vi "BallShear_BallShear.vi"(8 "Check":bool, 10 "Speed":dbl, 11 "Selected Balls":dbl[][](array[numeric])) -> (0 "Ready":bool, 3 "Status":string)   [LabVIEW 2013]
panel:
  in  "Y Val":dbl
  in  "X Val":dbl
  out "Selected Balls 2":dbl[][](array[numeric])
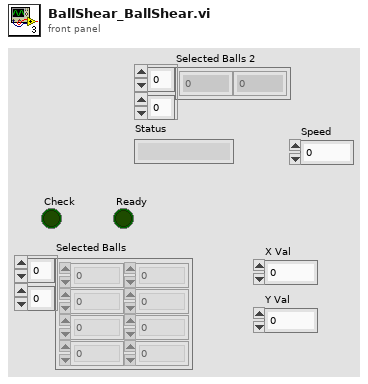
[diagram p1: front panel]
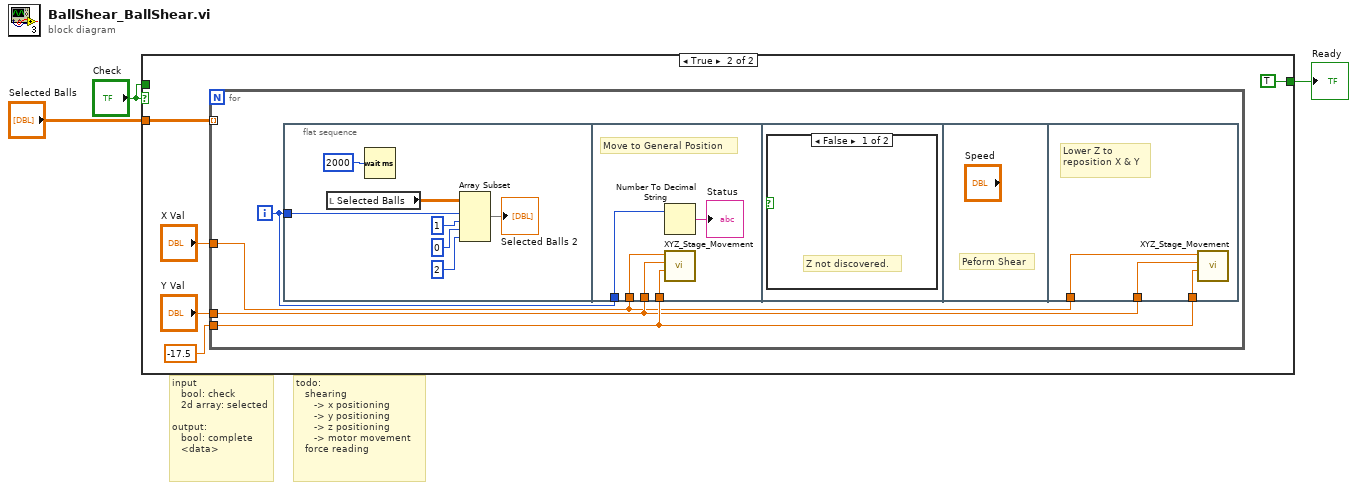
[diagram p0: block diagram]
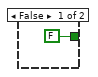
[diagram p2: hidden frame]
diagram:
  # "todo:\n   shearing\n      -> x positioning\n      -> y positioning\n      -> z positioning\n      -> motor movement\n   force reading"
  # "input\n   bool: check\n   2d array: selected\n\noutput:\n   bool: complete\n   <data>"
  n1 = case shown="True" "Check" {
    tunnel: "Check" -> [_ _]
    tunnel: [FALSE ("Power") TRUE ("Power")] -> w2
    tunnel: "Selected Balls" -> [_ w8]
    frame False {
    }
    frame True {
      n2 = for {
        tunnel: w8 -> [_] mode=indexing
        tunnel: -17.5 -> [w12]
        tunnel: "Y Val" -> [w11]
        tunnel: "X Val" -> [w10]
        i -> [w13]
        n3 = flat-sequence {
          tunnel: w13 -> [w15]
          tunnel: w13 -> [w25]
          tunnel: w12 -> [w23]
          tunnel: w11 -> [w22]
          tunnel: w10 -> [w21]
          tunnel: w12 -> [w28]
          tunnel: w11 -> [w27]
          tunnel: w10 -> [w26]
          frame #0 {
            n4 = local read "Selected Balls"() -> (w16:dbl[][])
            n5 = Wait (ms)(milliseconds to wait=u32 2000) -> ()  [unwired: 1 out]
            n6 = Array Subset(array=w16, index (row)=w15, length (row)=1 ("length"), index (col)=0 ("index"), length (col)=2 ("length")) -> (→"Selected Balls 2":dbl[][])
          }
          frame #1 {
            # "Move to General Position"
            n7 = Number To Decimal String(number=w25) -> (decimal integer string=→"Status":string)  [unwired: 1 in]
            n8 = call "XYZ_Stage_Movement.vi"("Z Input"=w23, "Y Input"=w22, "X Input"=w21) -> ()  [unwired: 6 in, 3 out]
          }
          frame #2 {
            n9 = case shown="False" {
              selector: _ -> [_ _]
              frame False {
                # "Z not discovered."
              }
              frame True {
                # "Previous Z from jog"
              }
            }
          }
          frame #3 {
            # "Peform Shear"
          }
          frame #4 {
            # "Lower Z to \nreposition X & Y"
            n10 = call "XYZ_Stage_Movement.vi"("Z Input"=w28, "Y Input"=w27, "X Input"=w26) -> ()  [unwired: 6 in, 3 out]
          }
        }
      }
    }
  }
  "Ready" <- w2
